vi "U16 Check.vi"(7 "16-bit array":bool[](array[boolean])=[FALSE, FALSE, FALSE, FALSE, FALSE, FALSE, FALSE, FALSE, FALSE, FALSE, FALSE, FALSE, FALSE, FALSE, FALSE, FALSE]) -> (6 "Lower Half has one?":bool, 8 "Half with one?":bool[](array[boolean]))   [LabVIEW 2011]
doc: "This VI splits 16-bit array and returns the half which contains a one"
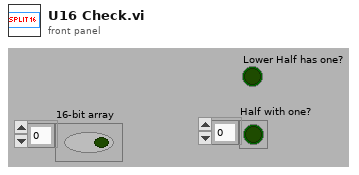
[diagram p1: front panel]
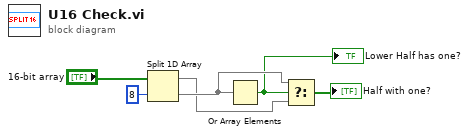
[diagram p0: block diagram]
diagram:
  n1 = Split 1D Array(array="16-bit array", index=8) -> (first subarray=w2:bool[], second subarray=w6:bool[])
  n2 = Or Array Elements(Boolean array=w6) -> (logical OR=w4:bool)
  "Lower Half has one?" <- w4
  n3 = Select(t=w6, s=w4, f=w2) -> (s? t:f=→"Half with one?":bool[])
